vi "Sift Initialize.vi"(6 "error in":errorcluster, 7 "API Key":string, 8 "API REST URL":string, 9 "API gRPC URL":string) -> (0 "error out":errorcluster, 3 "Sift Client out":refnum<class "Sift Client.lvclass">)   [LabVIEW 2024, in "Sift Stream.lvlib" / "Sift Stream.lvclass"]
doc: "Initialize Sift client and connection to Sift Proxy"
uses:
  Sift Stream.lvclass
  <vilib>/Sift/Sift/Sift API/Sift Client.lvclass
  Log Event Types.ctl
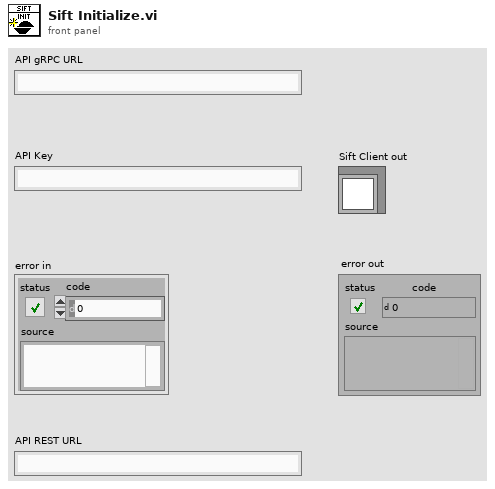
[diagram p1: front panel]
types:
  T1 = typedef "Sift Stream.lvlib/Sift Stream.lvclass/Log Event Types.ctl" = enum16{"INFO", "WARN", "ERROR"}
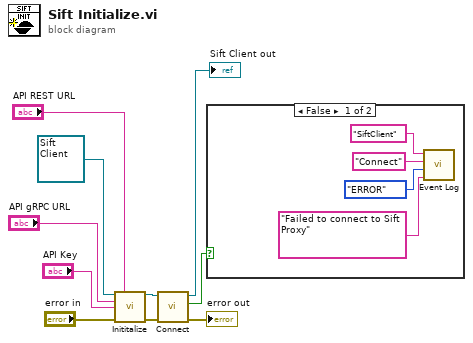
[diagram p0: block diagram]
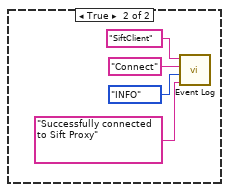
[diagram p2: hidden frame]
diagram:
  n1 = call-dynamic "Inititalize.vi"("Sift Client in"=refnum<class "Sift Client.lvclass"> refnum ("Sift Client.lvlib:Sift Client.lvclass"), "REST URL"="API REST URL", "GRPC URL"="API gRPC URL", "API Key"="API Key", "error in (no error)"="error in") -> ("Sift Client out"=w10:refnum<class "Sift Client.lvclass">, "error out"=w9:errorcluster)  [unwired: 9 in]
  n2 = call-dynamic "Connect.vi"("error in (no error)"=w9, "Sift Client in"=w10) -> ("error out"=→"error out":errorcluster, "Success"=w1:bool, "Sift Client out"=→"Sift Client out":refnum<class "Sift Client.lvclass">)  [unwired: 7 in]
  n3 = case shown="False" w1 {
    frame False {
      n4 = call "Event Log.vi"("Message"="Failed to connect to Sift Proxy", "Log Event Type"=Log_Event_Types."ERROR" ("Log Event Types"), "Event Type"="Connect", "Location"="SiftClient") -> ()  [unwired: 8 in]
    }
    frame True {
      n5 = call "Event Log.vi"("Message"="Successfully connected to Sift Proxy", "Log Event Type"=Log_Event_Types."INFO" ("Log Event Types"), "Event Type"="Connect", "Location"="SiftClient") -> ()  [unwired: 8 in]
    }
  }
